vi "CS++DMM-Triggered-Readout.vi"() -> ()   [LabVIEW 2016, in "CS++DMM.lvlib"]
uses:
  CS++DMM.lvlib
  CSPP_Core/Classes/CS++BaseClasses/Factory/CS++Factory.lvclass
  CS++DMM.lvclass
  C:/User/Brand/LVP/CSPP-Dev/Packages/CSPP_Core/Actors/CS++DeviceActor/CS++DeviceActor.lvclass
  CSPP_Core/Classes/CS++BaseClasses/Factory/CS++Factory.lvclass/CS++Factory.ctl
  CSPP_Core/Actors/CS++DeviceActor/CS++DeviceActor.lvclass/CS++DeviceActor.ctl
  CSPP_Core/Actors/CS++DeviceActor/Read Resource Name.vi
  CSPP_Core/Actors/CS++DeviceActor/CS++DeviceActor.lvclass
panel:
  out "dt":dbl[unit] format="%.3f"
  out "Nof points":i32 caption="actual number of points"
  out "Aperture":dbl[unit]
  in  "Device Index":i32
  out "Graph":dbl[](graph)
  in  "sample count":i32=10 caption="sample count (1)"
  in  "sample interval":dbl[unit]=0.1 caption="sample interval (0.0 s)" format="%.3f"
  in  "CS++Object Names":string[](array[string])=["DMM3458A-GPIB0-21", "DMM3458A-GPIB0-22"]
  in  "File Path Control":path=path "C:/User/Brand/LVP/STF/STF.ini"
  out "error out":errorcluster
  in  "Stop":bool
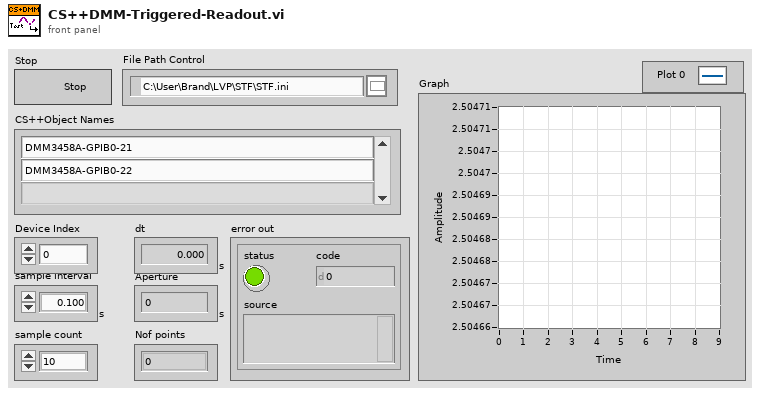
[diagram p1: front panel]
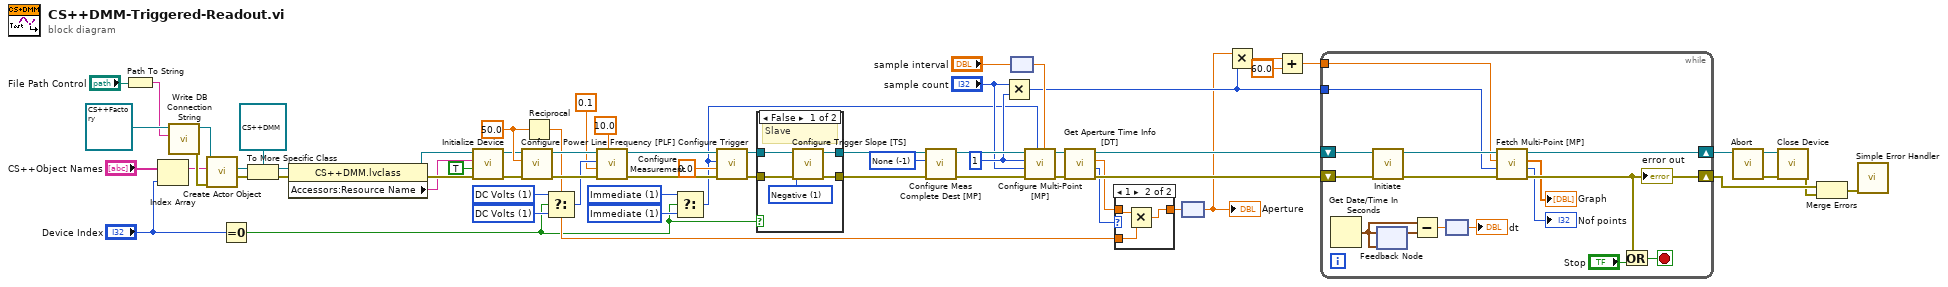
[diagram p0: block diagram]
diagram:
  w33 = -1 items=["None"=-1, "External"=2, "PXI TRIG0 or VXI TTL0"=111, "PXI TRIG1 or VXI TTL1"=112, "PXI TRIG2 or VXI TTL2"=113, "PXI TRIG3 or VXI TTL3"=114, "PXI TRIG4 or VXI TTL4"=115, "PXI TRIG5 or VXI TTL5"=116, "PXI TRIG6 or VXI TTL6"=117, "PXI TRIG7 or VXI TTL7"=118, "ECL0"=119, "ECL1"=120, "PXI Star"=131, "RTSI 0"=140, "RTSI 1"=141, "RTSI 2"=142, "RTSI 3"=143, "RTSI 4"=144, "RTSI 5"=145, "RTSI 6"=146] ("meas complete dest (None)")
  w34 = 1 items=["Immediate"=1, "External"=2, "Software Trigger Function"=3, "Interval"=10, "PXI TRIG0 or VXI TTL0"=111, "PXI TRIG1 or VXI TTL1"=112, "PXI TRIG2 or VXI TTL2"=113, "PXI TRIG3 or VXI TTL3"=114, "PXI TRIG4 or VXI TTL4"=115, "PXI TRIG5 or VXI TTL5"=116, "PXI TRIG6 or VXI TTL6"=117, "PXI TRIG7 or VXI TTL7"=118, "ECL0"=119, "ECL1"=120, "PXI Star"=131, "RTSI 0"=140, "RTSI 1"=141, "RTSI 2"=142, "RTSI 3"=143, "RTSI 4"=144, "RTSI 5"=145, "RTSI 6"=146] ("sample trigger (Immediate)")
  w35 = 1 items=["Immediate"=1, "External"=2, "Software Trigger Function"=3, "Interval"=10, "PXI TRIG0 or VXI TTL0"=111, "PXI TRIG1 or VXI TTL1"=112, "PXI TRIG2 or VXI TTL2"=113, "PXI TRIG3 or VXI TTL3"=114, "PXI TRIG4 or VXI TTL4"=115, "PXI TRIG5 or VXI TTL5"=116, "PXI TRIG6 or VXI TTL6"=117, "PXI TRIG7 or VXI TTL7"=118, "ECL0"=119, "ECL1"=120, "PXI Star"=131, "RTSI 0"=140, "RTSI 1"=141, "RTSI 2"=142, "RTSI 3"=143, "RTSI 4"=144, "RTSI 5"=145, "RTSI 6"=146] ("sample trigger (Immediate)")
  w12 = 1 ("trigger count (1)")
  w36 = 1 items=["DC Volts"=1, "AC Volts"=2, "DC Current"=3, "AC Current"=4, "2 Wire Resistance"=5, "4 Wire Resistance"=101, "AC + DC Volts"=106, "AC + DC Current"=107, "Frequency"=104, "Period"=105, "Temperature"=108] ("measurement function (DC Volts)")
  w38 = 1 items=["DC Volts"=1, "AC Volts"=2, "DC Current"=3, "AC Current"=4, "2 Wire Resistance"=5, "4 Wire Resistance"=101, "AC + DC Volts"=106, "AC + DC Current"=107, "Frequency"=104, "Period"=105, "Temperature"=108] ("measurement function (DC Volts)")
  w29 = 50.0 ("power line frequency (60.0 Hz)")
  n1 = Path To String(path="File Path Control") -> (string=w59:string)
  n2 = Index Array(array="CS++Object Names", index="Device Index") -> (element=w50:string)
  n3 = call "Write DB Connection String.vi"("DB Connection String"=w59, "CS++Factory in"=refnum<class "CS++Factory.lvclass"> refnum ("CS++BaseClasses.lvlib:CS++Factory.lvclass")) -> ("error out"=w54:errorcluster, "CS++Factory out"=w61:refnum<class "CS++Factory.lvclass">)  [unwired: 8 in]
  n4 = call "Create Actor Object.vi"("error in (no error)"=w54, "Object Name"=w50, "CS++Factory in"=w61) -> ("error out"=w48:errorcluster, "CS++BaseActor"=w49:refnum<class "CS++BaseActor.lvclass">)  [unwired: 5 in, 2 out]
  n5 = Equal To 0?(x="Device Index") -> (x = 0?=w25:bool)
  n6 = To More Specific Class(target class=refnum<class "CS++DMM.lvclass"> refnum ("CS++DMM.lvlib:CS++DMM.lvclass"), reference=w49, error in=w48) -> (specific class reference=w46:refnum<class "CS++DMM.lvclass">, error out=w44:errorcluster)
  n7 = property class="CS++DMM.lvclass"(reference=w46, error in=w44) -> (reference out=w45:refnum<class "CS++DMM.lvclass">, error out=w43:errorcluster, "Accessors:Resource Name"=w42:string)
  n8 = call "Initialize Device.vi"("error in (no error)"=w43, "Reset (F)"=TRUE, "Resource Name"=w42, "CS++DeviceActor in"=w45) -> ("error out"=w4:errorcluster, "CS++DeviceActor out"=w5:refnum<class "CS++DMM.lvclass">)  [unwired: 6 in]
  n9 = call "Configure Power Line Frequency [PLF].vi"("error in (no error)"=w4, "power line frequency (60.0 Hz)"=w29, "CS++DMM in"=w5) -> ("error out"=w39:errorcluster, "CS++DMM out"=w40:refnum<class "CS++DMM.lvclass">)  [unwired: 7 in]
  n10 = Reciprocal(x=w29) -> (1/x=w28:dbl)
  n11 = Select(t=w38, s=w25, f=w36) -> (s? t:f=w37:i32)
  n12 = call "Configure Measurement.vi"("range (-1.0: Auto)"=10.0, "error in (no error)"=w39, "absolute resolution (0.001)"=0.1, "measurement function (DC Volts)"=w37, "CS++DMM in"=w40) -> ("error out"=w20:errorcluster, "CS++DMM out"=w21:refnum<class "CS++DMM.lvclass">)  [unwired: 5 in]
  n13 = Select(t=w35, s=w25, f=w34) -> (s? t:f=w1:i32)
  n14 = call "Configure Trigger.vi"("error in (no error)"=w20, "trigger delay (0.0 s)"=0.0, "trigger source (Immediate)"=w1, "CS++DMM in"=w21) -> ("error out"=w23:errorcluster, "CS++DMM out"=w24:refnum<class "CS++DMM.lvclass">)  [unwired: 6 in]
  n15 = case shown="False" w25 {
    tunnel: w24 -> [w69 w71]
    tunnel: [w68 w71] -> w27
    tunnel: w23 -> [w67 w70]
    tunnel: [w66 w70] -> w26
    frame False {
      w65 = 1 items=["Positive", "Negative"] ("trigger slope (0: Positive)")
      # "Slave"
      n16 = call "Configure Trigger Slope [TS].vi"("error in (no error)"=w67, "trigger slope (0: Positive)"=w65, "CS++DMM in"=w69) -> ("error out"=w66:errorcluster, "CS++DMM out"=w68:refnum<class "CS++DMM.lvclass">)  [unwired: 7 in]
    }
    frame True {
      # "Master"
    }
  }
  n17 = call "Configure Meas Complete Dest [MP].vi"("error in (no error)"=w26, "meas complete dest (None)"=w33, "CS++DMM in"=w27) -> ("error out"=w18:errorcluster, "CS++DMM out"=w19:refnum<class "CS++DMM.lvclass">)  [unwired: 7 in]
  n18 = Multiply(x="sample count", y=w12) -> (x*y=w13:i32)
  n19 = node("sample interval") -> (w14:dbl)
  n20 = call "Configure Multi-Point [MP].vi"("sample interval (0.0 s)"=w14, "sample trigger (Immediate)"=w1, "error in (no error)"=w18, "sample count (1)"="sample count", "trigger count (1)"=w12, "CS++DMM in"=w19) -> ("error out"=w16:errorcluster, "CS++DMM out"=w17:refnum<class "CS++DMM.lvclass">)  [unwired: 4 in]
  n21 = call "Get Aperture Time Info [DT].vi"("error in (no error)"=w16, "CS++DMM in"=w17) -> ("error out"=w63:errorcluster, "aperture time units"=w32:i32, "aperture time (sec)"=w31:dbl, "CS++DMM out"=w64:refnum<class "CS++DMM.lvclass">)  [unwired: 6 in]
  n22 = case shown="1" w32 {
    tunnel: w31 -> [w72 w75]
    tunnel: [w72 w73] -> w30
    tunnel: w28 -> [_ w74]
    frame 0, Default {
    }
    frame 1 {
      n23 = Multiply(x=w75, y=w74) -> (x*y=w73:dbl)
    }
  }
  n24 = node(w30) -> (w6:dbl[unit])
  "Aperture" <- w6
  n25 = Multiply(x=w6, y=w13) -> (x*y=w53:dbl[unit])
  n26 = Add(x=w53, y=dbl[unit] 60.0 ("x")) -> (x+y=w51:dbl[unit])
  n27 = while {
    shift-right: [w86] -> w58
    shift-left: w63 -> [w78]
    shift-right: [w90] -> w10
    shift-left: w64 -> [w79]
    tunnel: w51 -> [w77]
    tunnel: w13 -> [w88]
    stop <- w87 stop-if-true
    n28 = Get Date/Time In Seconds() -> (seconds since 1Jan1904=w83:timestamp)
    n29 = call "Initiate.vi"("error in (no error)"=w78, "CS++DMM in"=w79) -> ("error out"=w76:errorcluster, "CS++DMM out"=w89:refnum<class "CS++DMM.lvclass">)  [unwired: 8 in]
    n30 = feedback-in #1(w83) -> ()
    n31 = feedback #1(w83) -> (w82:timestamp)
    n32 = Subtract(x=w83, y=w82) -> (x-y=w81:dbl)
    n33 = node(w81) -> (→"dt":dbl[unit])
    n34 = call "Fetch Multi-Point [MP].vi"("error in (no error)"=w76, "array size"=w88, "maximum time (5s)"=w77, "CS++DMM in"=w89) -> ("error out"=w86:errorcluster, "actual number of points"=→"Nof points":i32, "reading array"=→"Graph":dbl[], "CS++DMM out"=w90:refnum<class "CS++DMM.lvclass">)  [unwired: 4 in]
    "error out" <- w86
    n35 = Or(x=w86, y="Stop") -> (x .or. y?=w87:bool)
  }
  n36 = call "Abort.vi"("CS++DMM in"=w10) -> ("error out"=w8:errorcluster, "CS++DMM out"=w9:refnum<class "CS++DMM.lvclass">)  [unwired: 9 in]
  n37 = call "Close Device.vi"("error in (no error)"=w8, "CS++DeviceActor in"=w9) -> ("error out"=w57:errorcluster)  [unwired: 8 in, 1 out]
  n38 = Merge Errors(w58, w57) -> (w56:errorcluster)
  n39 = call <vilib>:"Simple Error Handler.vi"("error in (no error)"=w56) -> ()  [unwired: 4 in, 5 out]
